vi "Query controller status.vi"() -> ()   [LabVIEW 2016, in "Drivers.lvlib" / "Agilis.lvlib"]
uses:
  Agilis.lvlib
  Axis Status.ctl
  Limit Status.ctl
panel:
  out "Limit Status":T1[](array[typedef]) items=["Both inactive", "Ch1 active", "Ch2 active", "Both active"]
  out "Axis Status":T2[](array[typedef]) items=["Ready", "Stepping", "Jogging", "Moving to limit"]
  in  "Port":refnum<visa-resource-name>
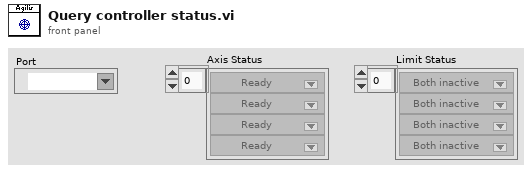
[diagram p1: front panel]
types:
  T1 = typedef "Drivers.lvlib/Agilis.lvlib/Limit Status.ctl" = i32
  T2 = typedef "Drivers.lvlib/Agilis.lvlib/Axis Status.ctl" = i32
  T3 = typedef "Drivers.lvlib/Agilis.lvlib/AgilisCmdLib Refnum.ctl" = refnum<k24>
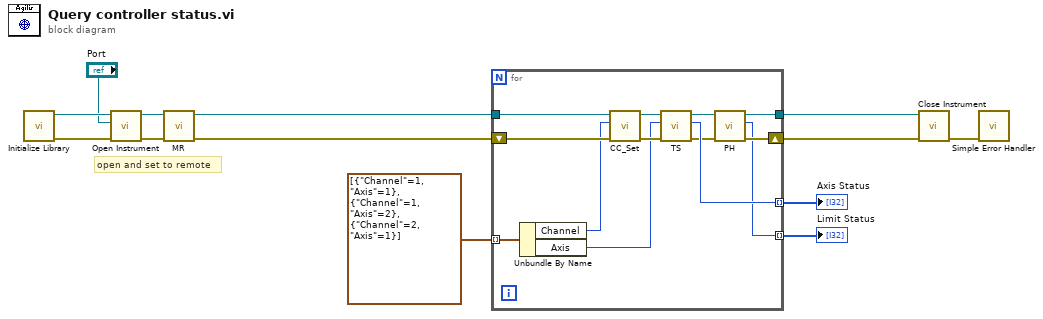
[diagram p0: block diagram]
diagram:
  # "open and set to remote"
  n1 = call "Initialize Library.vi"() -> ("error out"=w12:errorcluster, "Agilis out"=w13:T3)  [unwired: 10 in]
  n2 = call "Open Instrument.vi"("error in (no error)"=w12, "Device Key"="Port", "Agilis in"=w13) -> ("error out"=w5:errorcluster, "Agilis out"=w6:T3)  [unwired: 7 in]
  n3 = call "MR.vi"("error in (no error)"=w5, "Agilis in"=w6) -> ("error out"=w11:errorcluster, "Agilis out"=w4:T3)  [unwired: 8 in]
  n4 = for {
    tunnel: cluster{"Channel":i32, "Axis":i32}[] [{"Channel"=1, "Axis"=1}, {"Channel"=1, "Axis"=2}, {"Channel"=2, "Axis"=1}] -> [w26] mode=indexing
    tunnel: w4 -> [w25]
    shift-right: [w15] -> w8
    shift-left: w11 -> [w24]
    tunnel: [w17] -> w3
    tunnel: [w19] -> w2 mode=indexing
    tunnel: [w14] -> w1 mode=indexing
    n5 = Unbundle By Name(w26) -> ("Channel"=w23:i32, "Axis"=w20:i32)
    n6 = call "CC_Set.vi"("error in (no error)"=w24, "Channel Number"=w23, "Agilis in"=w25) -> ("error out"=w21:errorcluster, "Agilis out"=w22:T3)  [unwired: 7 in]
    n7 = call "TS.vi"("error in (no error)"=w21, "Axis Number"=w20, "Agilis in"=w22) -> ("error out"=w16:errorcluster, "Axis Status"=w19:T2, "Agilis out"=w18:T3)  [unwired: 6 in]
    n8 = call "PH.vi"("error in (no error)"=w16, "Agilis in"=w18) -> ("error out"=w15:errorcluster, "Limit Status"=w14:T1, "Agilis out"=w17:T3)  [unwired: 7 in]
  }
  "Axis Status" <- w2
  "Limit Status" <- w1
  n9 = call "Close Instrument.vi"("error in (no error)"=w8, "Agilis in"=w3) -> ("error out"=w7:errorcluster)  [unwired: 9 in]
  n10 = call <vilib>:"Simple Error Handler.vi"("error in (no error)"=w7) -> ()  [unwired: 4 in, 5 out]
